vi "Find-Classes.vi"() -> ()   [LabVIEW 2016]
uses:
  MongoDB-Driver/MongoDB-Client/MongoDB-Client/MongoDB-Client.lvclass
  MongoDB-Driver/MongoDB-Database/MongoDB-Database/MongoDB-Database.lvclass
  MongoDB-Driver/MongoDB-Collection/MongoDB-Collection/MongoDB-Collection.lvclass
  HITRAN-Line-Cluster.ctl
panel:
  out "#Lines":i32
  out "Casting Time (ms)":u32
  out "Selection Time (ms)":u32
  out "Lines":T1[](array[typedef])
  out "GetNumberOfDocs":i64
  out "ListCollections":string[](array[string])
  out "ListDatabases":string[](array[string])
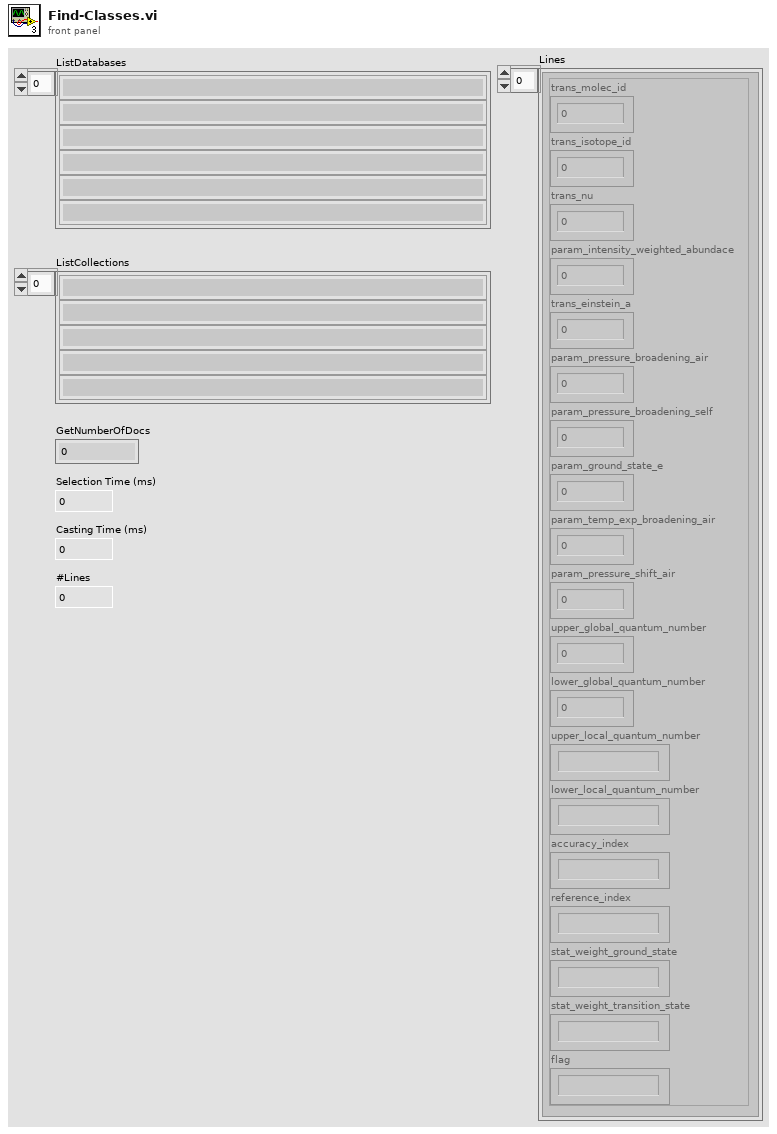
[diagram p1: front panel]
types:
  T1 = typedef "HITRAN-Line-Cluster.ctl" = cluster{"trans_molec_id":i32, "trans_isotope_id":i32, "trans_nu":dbl, "param_intensity_weighted_abundace":dbl, "trans_einstein_a":dbl, "param_pressure_broadening_air":dbl, "param_pressure_broadening_self":dbl, "param_ground_state_e":dbl, "param_temp_exp_broadening_air":dbl, "param_pressure_shift_air":dbl, "upper_global_quantum_number":i32, "lower_global_quantum_number":i32, "upper_local_quantum_number":string, "lower_local_quantum_number":string, "accuracy_index":string, "reference_index":string, "stat_weight_ground_state":string, "stat_weight_transition_state":string, "flag":string}
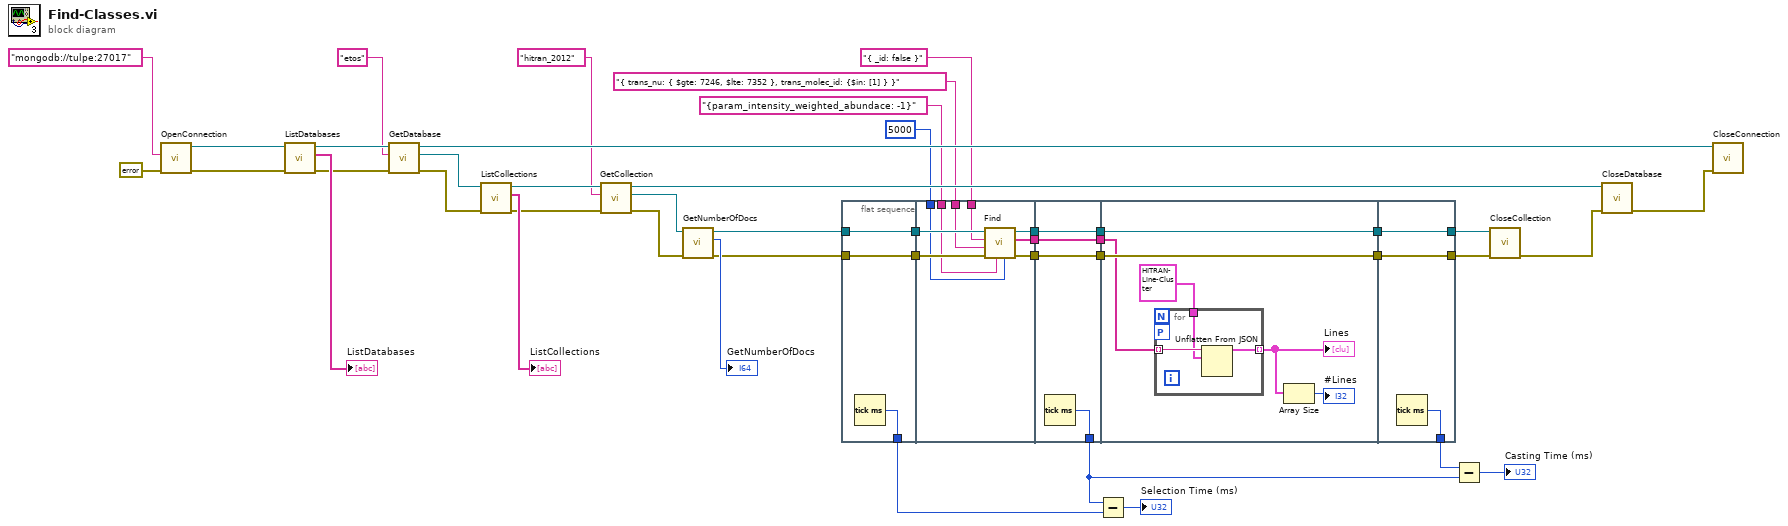
[diagram p0: block diagram]
diagram:
  n1 = call "OpenConnection.vi"("error in (no error)"=errorcluster {"status"=FALSE, "code"=0, "source"=""}, "MongoDB Connection String"="mongodb://tulpe:27017" ("connectionString")) -> ("error out"=w41:errorcluster, "MongoDB-Client out"=w42:refnum<class "MongoDB-Client.lvclass">)  [unwired: 8 in]
  n2 = call "ListDatabases.vi"("error in (no error)"=w41, "MongoDB-Client in"=w42) -> ("error out"=w38:errorcluster, "ListDatabases"=→"ListDatabases":string[], "MongoDB-Client out"=w39:refnum<class "MongoDB-Client.lvclass">)  [unwired: 7 in]
  n3 = call "GetDatabase.vi"("error in (no error)"=w38, "databaseName"="etos" ("connectionString"), "MongoDB-Client in"=w39) -> ("error out"=w34:errorcluster, "MongoDB-Database"=w35:refnum<class "MongoDB-Database.lvclass">, "MongoDB-Client out"=w36:refnum<class "MongoDB-Client.lvclass">)  [unwired: 6 in]
  n4 = call "ListCollections.vi"("error in (no error)"=w34, "MongoDB-Database in"=w35) -> ("error out"=w31:errorcluster, "ListCollections"=→"ListCollections":string[], "MongoDB-Database out"=w32:refnum<class "MongoDB-Database.lvclass">)  [unwired: 7 in]
  n5 = call "GetCollection.vi"("error in (no error)"=w31, "collectionName"="hitran_2012" ("connectionString"), "MongoDB-Database in"=w32) -> ("error out"=w25:errorcluster, "MongoDB-Collection"=w26:refnum<class "MongoDB-Collection.lvclass">, "MongoDB-Database out"=w29:refnum<class "MongoDB-Database.lvclass">)  [unwired: 6 in]
  n6 = call "GetNumberOfDocs.vi"("error in (no error)"=w25, "MongoDB-Collection in"=w26) -> ("error out"=w20:errorcluster, "GetNumberOfDocs"=→"GetNumberOfDocs":i64, "MongoDB-Collection out"=w23:refnum<class "MongoDB-Collection.lvclass">)  [unwired: 7 in]
  n7 = flat-sequence {
    tunnel: w20 -> [w46]
    tunnel: w23 -> [w47]
    tunnel: [w47] -> w16
    tunnel: [w46] -> w15
    tunnel: [w45] -> w6
    tunnel: "{ _id: false }" ("selectionString") -> [w55]
    tunnel: "{ trans_nu: { $gte: 7246, $lte: 7352 }, trans_molec_id: {$in: [1] } }" ("filterString") -> [w54]
    tunnel: "{param_intensity_weighted_abundace: -1}" ("sortString") -> [w48]
    tunnel: 5000 ("limitInteger") -> [w52]
    tunnel: w16 -> [w56]
    tunnel: w15 -> [w53]
    tunnel: [w51] -> w14
    tunnel: [w50] -> w13
    tunnel: [w49] -> w12
    tunnel: w14 -> [w60]
    tunnel: w13 -> [w59]
    tunnel: w12 -> [w58]
    tunnel: [w57] -> w2
    tunnel: [w60] -> w11
    tunnel: [w59] -> w10
    tunnel: [w58] -> w9
    tunnel: w11 -> [w66]
    tunnel: w10 -> [w65]
    tunnel: w9 -> [w63]
    tunnel: [w66] -> w8
    tunnel: [w65] -> w7
    tunnel: [w71] -> w17
    tunnel: [w72] -> w18
    tunnel: w8 -> [w72]
    tunnel: w7 -> [w71]
    tunnel: [w70] -> w5
    frame #0 {
      n8 = Tick Count (ms)() -> (millisecond timer value=w45:u32)
    }
    frame #1 {
      n9 = call "Find.vi"("limitInteger"=w52, "sortString"=w48, "error in (no error)"=w53, "filterString"=w54, "selectionString"=w55, "MongoDB-Collection in"=w56) -> ("error out"=w50:errorcluster, "Find"=w49:string[], "MongoDB-Collection out"=w51:refnum<class "MongoDB-Collection.lvclass">)  [unwired: 3 in]
    }
    frame #2 {
      n10 = Tick Count (ms)() -> (millisecond timer value=w57:u32)
    }
    frame #3 {
      n11 = for {
        tunnel: T1 {"trans_molec_id"=0, "trans_isotope_id"=0, "trans_nu"=0.0, "param_intensity_weighted_abundace"=0.0, "trans_einstein_a"=0.0, "param_pressure_broadening_air"=0.0, "param_pressure_broadening_self"=0.0, "param_ground_state_e"=0.0, "param_temp_exp_broadening_air"=0.0, "param_pressure_shift_air"=0.0, "upper_global_quantum_number"=0, "lower_global_quantum_number"=0, "upper_local_quantum_number"="", "lower_local_quantum_number"="", "accuracy_index"="", "reference_index"="", "stat_weight_ground_state"="", "stat_weight_transition_state"="", "flag"=""} ("HITRAN-Line-Cluster") -> [w67]
        tunnel: [w69] -> w62 mode=indexing
        tunnel: w63 -> [w68] mode=indexing
        workers-P: _ -> [_]
        n12 = Unflatten From JSON(JSON string=w68, type and defaults=w67) -> (value=w69:T1)  [unwired: 5 in, 1 out]
      }
      "Lines" <- w62
      n13 = Array Size(array=w62) -> (size(s)=→"#Lines":i32)
    }
    frame #4 {
      n14 = Tick Count (ms)() -> (millisecond timer value=w70:u32)
    }
  }
  n15 = Subtract(x=w2, y=w6) -> (x-y=→"Selection Time (ms)":u32)
  n16 = Subtract(x=w5, y=w2) -> (x-y=→"Casting Time (ms)":u32)
  n17 = call "CloseCollection.vi"("error in (no error)"=w17, "MongoDB-Collection in"=w18) -> ("error out"=w27:errorcluster)  [unwired: 9 in]
  n18 = call "CloseDatabase.vi"("error in (no error)"=w27, "MongoDB-Database in"=w29) -> ("error out"=w28:errorcluster)  [unwired: 9 in]
  n19 = call "CloseConnection.vi"("error in (no error)"=w28, "MongoDB-Client in"=w36) -> ()  [unwired: 9 in, 1 out]
